vi "Clipborad Text.vi"() -> ()   [LabVIEW 2011]
panel:
  out "Waveform Chart 2":dbl(graph)
  out "Waveform Chart":dbl(graph)
  in  "stop":bool
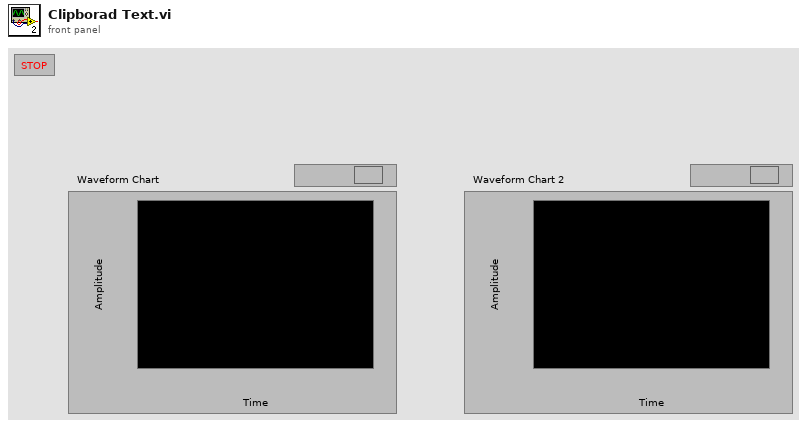
[diagram p1: front panel]
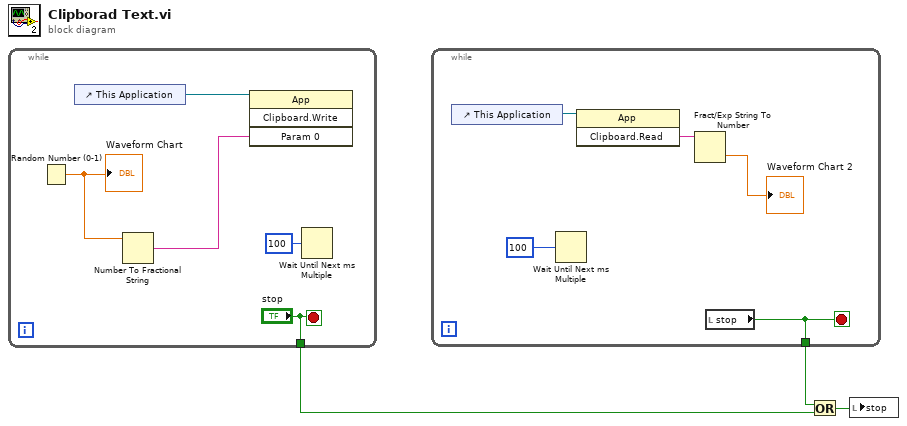
[diagram p0: block diagram]
diagram:
  n1 = while {
    tunnel: ["stop"] -> w1
    stop <- "stop" stop-if-true
    n2 = Random Number (0-1)() -> (number: 0 to 1=w8:dbl)
    "Waveform Chart" <- w8
    n3 = control-ref of="This Application"() -> (w7:refnum<vi>)
    n4 = Number To Fractional String(number=w8) -> (F-format string=w6:string)  [unwired: 3 in]
    n5 = invoke class="App" method="Clipboard.Write"(reference=w7, "Param 0"=w6) -> ()  [unwired: 2 in, 4 out]
    n6 = Wait Until Next ms Multiple(millisecond multiple=u32 100) -> ()  [unwired: 1 out]
  }
  n7 = while {
    tunnel: [w10] -> w2
    stop <- w10 stop-if-true
    n8 = control-ref of="This Application"() -> (w13:refnum<vi>)
    n9 = Wait Until Next ms Multiple(millisecond multiple=u32 100) -> ()  [unwired: 1 out]
    n10 = invoke class="App" method="Clipboard.Read"(reference=w13) -> ("Read Clipbrd"=w12:string)  [unwired: 2 in, 2 out]
    n11 = Fract/Exp String To Number(string=w12) -> (number=→"Waveform Chart 2":dbl)  [unwired: 3 in, 1 out]
    n12 = local read "stop"() -> (w10:bool)
  }
  n13 = Or(x=w2, y=w1) -> (x .or. y?=w3:bool)
  n14 = local write "stop"(w3) -> ()
